vi "GenericJoystickDeadband.vi"(2 "Deadband":dbl(slide) min=0.0 max=0.4 scale=0.0..0.4, 3 "Raw Joystick Value":dbl) -> (1 "Scaled Joystick Value":dbl)   [LabVIEW 2019]
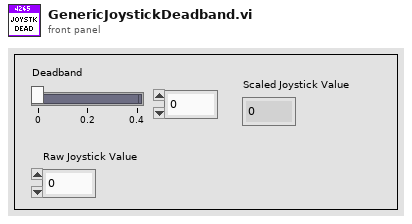
[diagram p1: front panel]
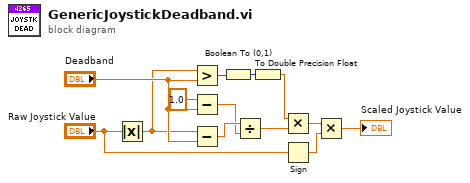
[diagram p0: block diagram]
diagram:
  n1 = Absolute Value(x="Raw Joystick Value") -> (abs(x)=w3:dbl)
  n2 = Greater?(x=w3, y="Deadband") -> (0:w2:bool)
  n3 = Subtract(x=1.0, y="Deadband") -> (x-y=w7:dbl)
  n4 = Subtract(x=w3, y="Deadband") -> (x-y=w9:dbl)
  n5 = Boolean To (0,1)(Boolean=w2) -> (0, 1=w11:i16)
  n6 = Divide(x=w9, y=w7) -> (x/y=w6:dbl)
  n7 = To Double Precision Float(number=w11) -> (double precision float=w10:dbl)
  n8 = Multiply(x=w10, y=w6) -> (x*y=w12:dbl)
  n9 = Sign(1:"Raw Joystick Value") -> (0:w4:dbl)
  n10 = Multiply(x=w12, y=w4) -> (x*y=→"Scaled Joystick Value":dbl)
